vi "PrimaryAttackerRole.vi"(8 "error in (no error)":errorcluster, 11 "PrimaryAttackerRole in":refnum<class "PrimaryAttackerRole.lvclass">) -> (0 "error out":errorcluster, 3 "PrimaryAttackerRole out":refnum<class "PrimaryAttackerRole.lvclass">)   [LabVIEW 2023, in "PrimaryAttackerRole.lvclass"]
uses:
  PrimaryAttackerRole.lvclass
  C:/Users/ebert/Documents/codes/SSL/repo/SSL_AI/Role_class/Role.lvclass
  Robot_class/Robot.lvclass
  Game_class/Game.lvclass
  Role_class/Role.lvclass/Role.ctl
  PrimaryAttackerRole_states.ctl
  ShootTactic_class/States.ctl
  Tacticbook_class/Tacticbook.lvclass/Tacticbook.ctl
  ShootTactic_class/ShootTactic.lvclass/ShootTactic.ctl
  Tacticbook_class/Read ShootTactic.vi
  ShootTactic_class/Read States.vi
  Tacticbook_class/Read TestTactic.vi
  Role_class/Read Tacticbook.vi
  Role_class/Write Tacticbook.vi
  Role_class/Write tactic_index.vi
  Role_class/Read RobotRef.vi
  Tacticbook_class/Tacticbook.lvclass
  ShootTactic_class/ShootTactic.lvclass
  TestTactic_class/TestTactic.lvclass
panel:
  out "Game out":refnum<class "Game.lvclass">
  in  "Game in":refnum<class "Game.lvclass">
  out "Robot out":refnum<class "Robot.lvclass">
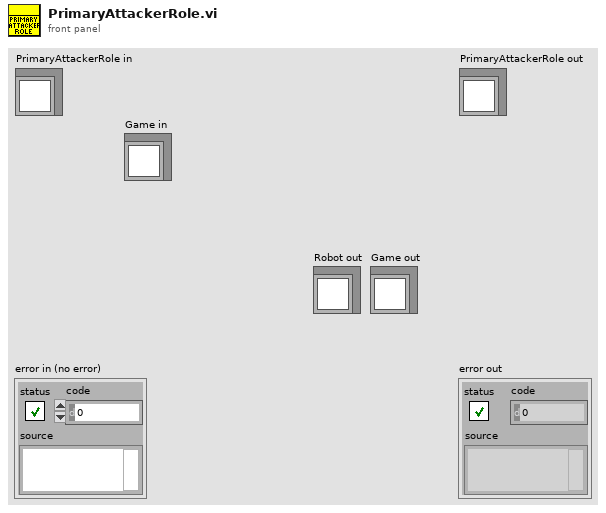
[diagram p1: front panel]
types:
  T1 = typedef "PrimaryAttackerRole.lvclass/PrimaryAttackerRole_states.ctl" = enum16{"Shoot", "PreparePass", "Pass", "Exit"}
  T2 = typedef "ShootTactic.lvclass/States.ctl" = enum16{"BallInGoalieArea", "Exit", "KickToGoal", "StealBall"}
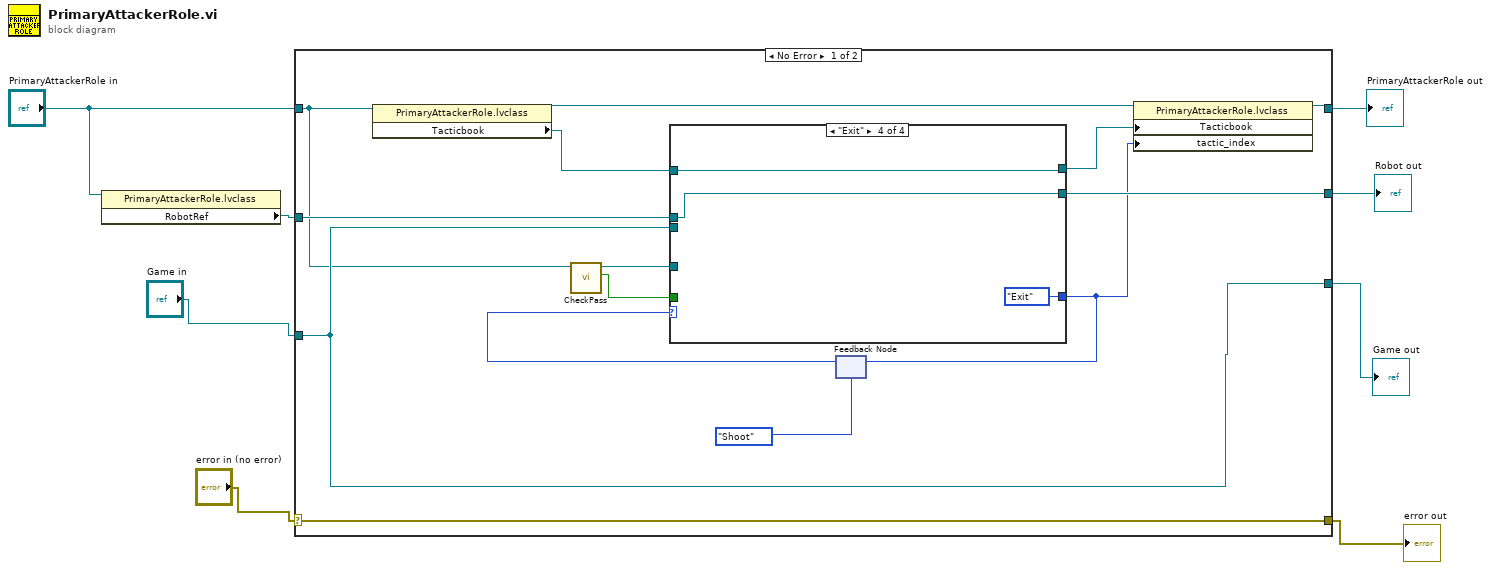
[diagram p0: block diagram]
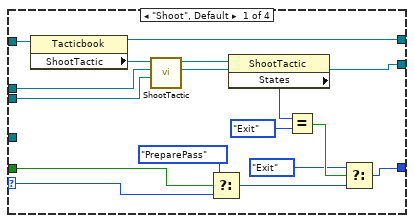
[diagram p2: hidden frame]
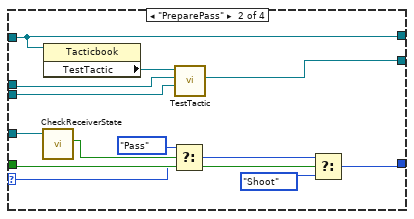
[diagram p3: hidden frame]
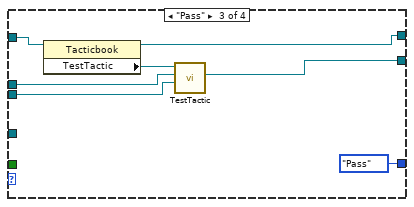
[diagram p4: hidden frame]
diagram:
  n1 = property class="PrimaryAttackerRole.lvclass"(reference="PrimaryAttackerRole in") -> ("RobotRef"=w5:refnum<class "Robot.lvclass">)  [unwired: 1 in, 2 out]
  n2 = case shown="No Error" "error in (no error)" {
    selector: "error in (no error)" -> [w22 w65]
    tunnel: [w22 w65] -> w3
    tunnel: [w21 w62] -> w2
    tunnel: w5 -> [w15 w64]
    tunnel: [w17 w64] -> w8
    tunnel: [w14 w63] -> w7
    tunnel: "Game in" -> [w14 w63]
    tunnel: "PrimaryAttackerRole in" -> [w12 w62]
    frame No Error {
      n3 = property class="PrimaryAttackerRole.lvclass"(reference=w12) -> (reference out=w20:refnum<class "PrimaryAttackerRole.lvclass">, "Tacticbook"=w18:refnum<class "Tacticbook.lvclass">)  [unwired: 1 in, 1 out]
      n4 = call-dynamic "CheckPass.vi"("object in"=w12) -> ("pass"=w11:bool, "object out"=w10:refnum<class "PrimaryAttackerRole.lvclass">)  [unwired: 8 in, 1 out]
      n5 = feedback #1(PrimaryAttackerRole_states."Shoot" ("Enum")) -> (w19:T1)
      n6 = case shown="\"Exit\"" w19 {
        selector: w19 -> [w24 w42 _ _]
        tunnel: [w36 w41 PrimaryAttackerRole_states."Pass" ("f") PrimaryAttackerRole_states."Exit" ("f")] -> w9
        tunnel: w18 -> [w38 w49 w56 w60]
        tunnel: w15 -> [w34 w47 w55 w59]
        tunnel: [w32 w45 w53 w59] -> w17
        tunnel: [w28 w49 w52 w60] -> w16
        tunnel: w14 -> [w33 w46 w54 _]
        tunnel: w11 -> [w23 w51 _ _]
        tunnel: w10 -> [_ w40 _ _]
        frame "Shoot", Default {
          n7 = property class="Tacticbook"(reference=w38) -> (reference out=w28:refnum<class "Tacticbook.lvclass">, "ShootTactic"=w35:refnum<class "ShootTactic.lvclass">)  [unwired: 1 in, 1 out]
          n8 = call "ShootTactic.vi"("Game in"=w33, "Robot"=w34, "ShootTactic in"=w35) -> ("Robot out"=w32:refnum<class "Robot.lvclass">, "ShootTactic out"=w31:refnum<class "ShootTactic.lvclass">)  [unwired: 5 in, 2 out]
          n9 = Select(t=PrimaryAttackerRole_states."PreparePass" ("Enum"), s=w23, f=w24) -> (s? t:f=w26:T1)
          n10 = property class="ShootTactic"(reference=w31) -> ("States"=w29:T2)  [unwired: 1 in, 2 out]
          n11 = Equal?(x=w29, y=States."Exit") -> (x = y?=w37:bool)
          n12 = Select(t=PrimaryAttackerRole_states."Exit" ("Enum"), s=w37, f=w26) -> (s? t:f=w36:T1)
        }
        frame "PreparePass" {
          n13 = call "CheckReceiverState.vi"("object in"=w40) -> ("pass"=w39:bool)  [unwired: 8 in, 2 out]
          n14 = property class="Tacticbook"(reference=w49) -> ("TestTactic"=w48:refnum<class "TestTactic.lvclass">)  [unwired: 1 in, 2 out]
          n15 = Select(t=PrimaryAttackerRole_states."Pass" ("f"), s=w39, f=w42) -> (s? t:f=w43:T1)
          n16 = call-dynamic "TestTactic.vi"("Game in"=w46, "Robot"=w47, "Tactic in"=w48) -> ("Robot out"=w45:refnum<class "Robot.lvclass">)  [unwired: 6 in, 2 out]
          n17 = Select(t=w43, s=w51, f=PrimaryAttackerRole_states."Shoot") -> (s? t:f=w41:T1)
        }
        frame "Pass" {
          n18 = property class="Tacticbook"(reference=w56) -> (reference out=w52:refnum<class "Tacticbook.lvclass">, "TestTactic"=w58:refnum<class "TestTactic.lvclass">)  [unwired: 1 in, 1 out]
          n19 = call-dynamic "TestTactic.vi"("Game in"=w54, "Robot"=w55, "Tactic in"=w58) -> ("Robot out"=w53:refnum<class "Robot.lvclass">)  [unwired: 6 in, 2 out]
        }
        frame "Exit" {
        }
      }
      n20 = feedback-in #1(w9) -> ()
      n21 = property class="PrimaryAttackerRole.lvclass"(reference=w20, "Tacticbook"=w16, "tactic_index"=w9) -> (reference out=w21:refnum<class "PrimaryAttackerRole.lvclass">)  [unwired: 1 in, 1 out]
    }
    frame Error {
    }
  }
  "error out" <- w3
  "PrimaryAttackerRole out" <- w2
  "Robot out" <- w8
  "Game out" <- w7
